vi "Run All.vi"(8 "Error In":errorcluster) -> (0 "Error Out":errorcluster)   [LabVIEW 2017, in "Tests.lvlib"]
uses:
  Tests.lvlib
  <vilib>/addons/_JKI Toolkits/Caraya/classes/Test/Test.lvclass
  Parser/Parser.lvlib
  Readers/Readers.lvlib
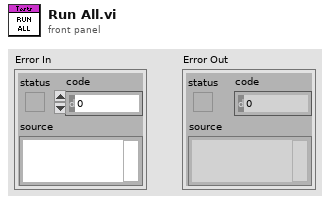
[diagram p1: front panel]
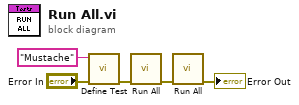
[diagram p0: block diagram]
diagram:
  n1 = call <vilib>:"Define Test.vi"("error in (no error)"="Error In", "Label (VI Title)"="Mustache") -> ("error out"=w2:errorcluster)  [unwired: 9 in]
  n2 = call "Run All.vi"("Error In"=w2) -> ("Error Out"=w1:errorcluster)  [unwired: 10 in]
  n3 = call "Run All.vi"("Error In"=w1) -> ("Error Out"=→"Error Out":errorcluster)  [unwired: 10 in]
